vi "Update New Selection.vi"(7 "Node ID":i32, 8 "error in (no error)":errorcluster, 9 "Shape in":refnum<data-value>[](array[refnum]), 10 "Selected in":i16[](array[numeric]), 11 "Image in":refnum<class "Image.lvclass">) -> (0 "error out":errorcluster, 1 "Shape out 2":refnum<data-value>[](array[refnum]), 2 "Selected out 2":i16[](array[numeric]), 3 "Image out":refnum<class "Image.lvclass">)   [LabVIEW 2017, in "LV Image Editor Framework.lvlib" / "Image Editor Handler.lvclass"]
uses:
  Image Editor Handler.lvclass
  Image/Image.lvclass
  Forms/Shape/Shape.lvclass
  Forms/Selection/Selection.lvclass
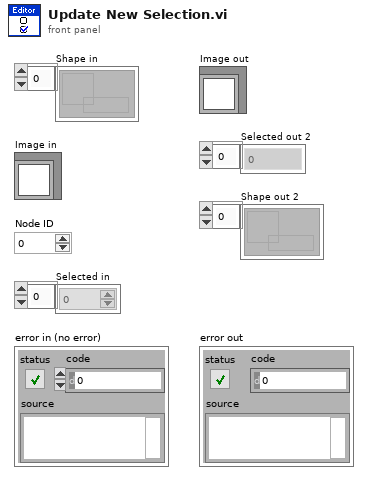
[diagram p1: front panel]
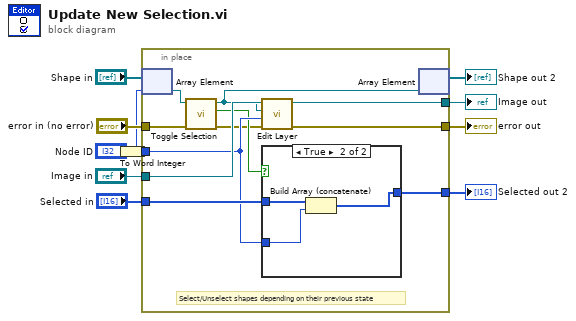
[diagram p0: block diagram]
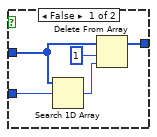
[diagram p2: hidden frame]
diagram:
  n1 = To Word Integer(number="Node ID") -> (16bit integer=w1:i16)
  n2 = in-place {
    in-place-border: [w11] -> w3
    in-place-border: "error in (no error)" -> [w20]
    in-place-border: "Image in" -> [w19]
    in-place-border: w1 -> [w15]
    in-place-border: [w17] -> w5
    in-place-border: "Selected in" -> [w16]
    in-place-border: [w14] -> w6
    # "Select/Unselect shapes depending on their previous state"
    n3 = in-place-array #1("Shape in", w1) -> (w21:refnum<data-value>)
    n4 = call "Toggle Selection.vi"("error in (no error)"=w20, "Shape"=w21) -> ("error out"=w12:errorcluster, "New State"=w13:bool, "Shape"=w18:refnum<data-value>)  [unwired: 7 in]
    n5 = call "Edit Layer.vi"("error in (no error)"=w12, "Layer Index"=w15, "ShapeRef"=w18, "Image in"=w19) -> ("error out"=w11:errorcluster, "Image out"=w17:refnum<class "Image.lvclass">)  [unwired: 6 in]
    n6 = case shown="True" w13 {
      tunnel: w16 -> [w22 w29]
      tunnel: w15 -> [w26 w28]
      tunnel: [w23 w27] -> w14
      frame False {
        n7 = Search 1D Array(1D array=w22, element=w26) -> (index of element=w25:i32)  [unwired: 1 in]
        n8 = Delete From Array(array=w22, length=1, index=w25) -> (array with subset deleted=w23:i16[])  [unwired: 1 out]
      }
      frame True {
        n9 = Build Array (concatenate)(w29, w28) -> (w27:i16[])
      }
    }
    n10 = in-place-array #1(w18) -> (→"Shape out 2":refnum<data-value>[])  [unwired: 1 out]
  }
  "Selected out 2" <- w6
  "Image out" <- w5
  "error out" <- w3
